vi "host.vi"() -> ()   [LabVIEW 2017]
panel:
  in  "Plot Color":u32(colorbox)=16715776
  in  "Grid Color":u32(colorbox)
  in  "Visible Section":u16(ring)=8
  out "Polar Plot":picture
  in  "stop":bool
  out "data":dbl(graph)
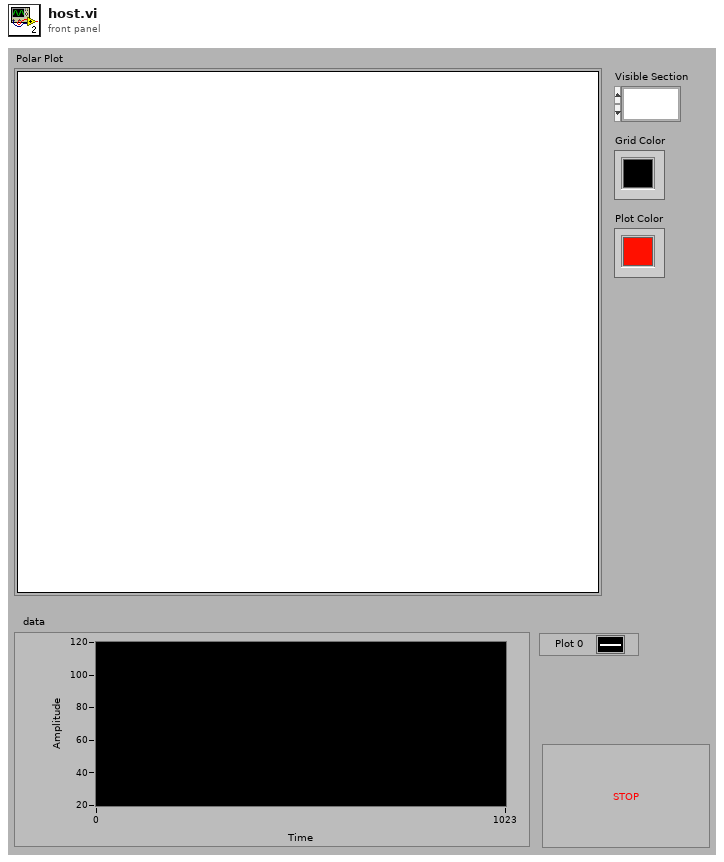
[diagram p1: front panel]
types:
  T1 = cluster{"maximum":dbl, "minimum":dbl, "clip to min":bool, "log?(F)":bool, "grid color":u32, "plot color":u32, "format and precision":cluster{"format":enum8{"Decimal", "Scientific", "Engineering", "Binary", "Octal", "Hex"}, "precision":u8}, "visible section":u16}
  T2 = typedef "LVBoundsTypeDef.ctl" = cluster{"Width":u32, "Height":u32}
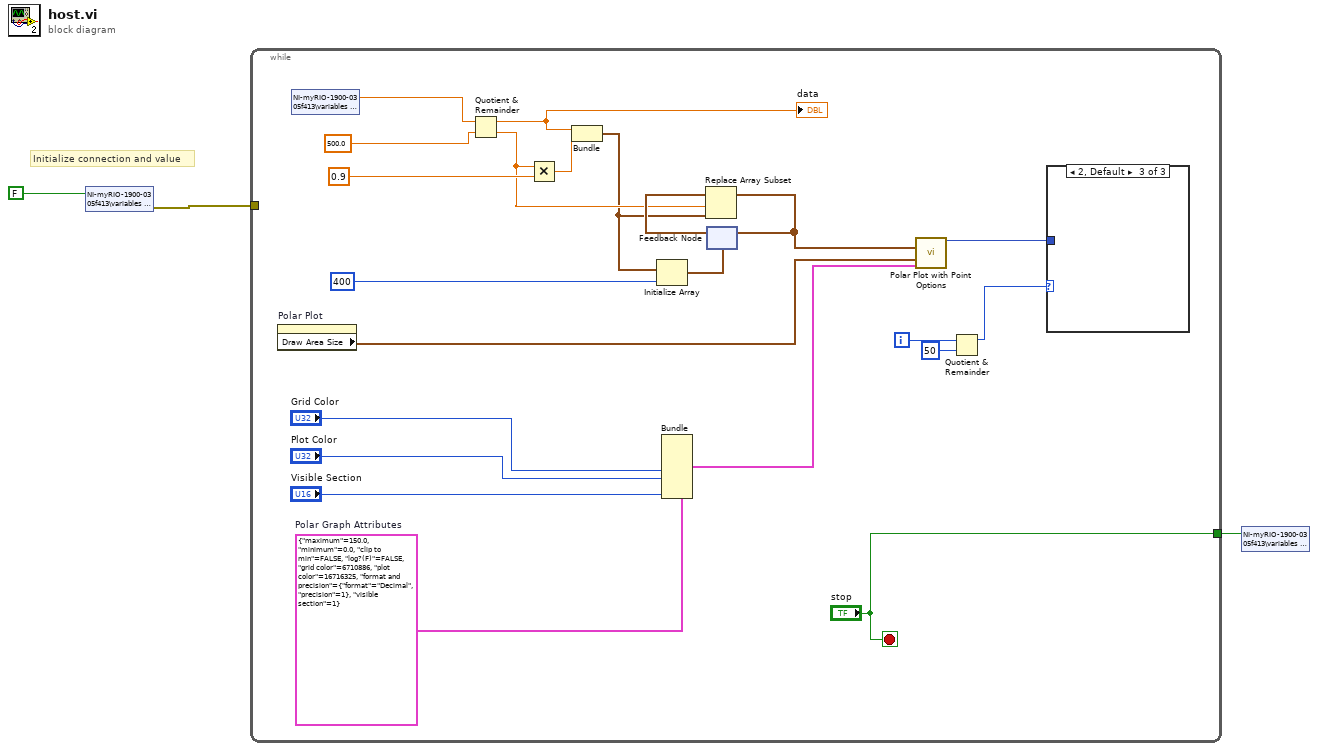
[diagram p0: block diagram]
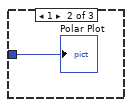
[diagram p3: hidden frame]
diagram:
  # "Initialize connection and value"
  n1 = shared-variable "NI-myRIO-1900-0305f413\\variables - network - RT.lvlib\\stop"(FALSE) -> (error out=w2:errorcluster)  [unwired: 1 in]
  n2 = while {
    tunnel: ["stop"] -> w3
    tunnel: w2 -> [_]
    i -> [w6]
    stop <- "stop" stop-if-true
    w11 = T1 {"maximum"=150.0, "minimum"=0.0, "clip to min"=FALSE, "log?(F)"=FALSE, "grid color"=6710886, "plot color"=16716325, "format and precision"={"format"=enum."Decimal", "precision"=1}, "visible section"=1}  # Polar Graph Attributes
    n3 = property on="Polar Plot" class="Pict"() -> ("Draw Area Size"=w22:T2)  [unwired: 2 in, 2 out]
    n4 = shared-variable "NI-myRIO-1900-0305f413\\variables - network - RT.lvlib\\data"() -> (w24:dbl)  [unwired: 1 in, 1 out]
    n5 = Quotient & Remainder(x=w24, y=500.0) -> (x-y*floor(x/y)=w15:dbl, floor(x/y)=w17:dbl)
    "data" <- w15
    n6 = Multiply(x=w17, y=0.9) -> (x*y=w19:dbl)
    n7 = Bundle(w15, w19) -> (w12:cluster{dbl, dbl})  [unwired: 1 in]
    n8 = Initialize Array(w12, 400 ("dimension size")) -> (w14:cluster{dbl, dbl}[])
    n9 = Bundle(cluster=w11, "grid color"="Grid Color", "plot color"="Plot Color", "visible section"="Visible Section") -> (w7:T1)  [unwired: 5 in]
    n10 = feedback #1(w14) -> (w18:cluster{dbl, dbl}[])
    n11 = Replace Array Subset(array=w18, new element=w12, index=w17) -> (w16:cluster{dbl, dbl}[])
    n12 = feedback-in #1(w16) -> ()
    n13 = call <vilib>:"Polar Plot with Point Options.vi"("data array [mag, phase (deg)]"=w16, "dimensions (w,h)"=w22, "polar attributes"=w7) -> ("new picture"=w21:picture)  [unwired: 12 in]
    n14 = Quotient & Remainder(x=w6, y=50) -> (x-y*floor(x/y)=w4:i32)  [unwired: 1 out]
    n15 = case shown="2, Default" w4 {
      tunnel: w21 -> [_ w26 _]
      frame 0 {
      }
      frame 1 {
        "Polar Plot" <- w26
      }
      frame 2, Default {
      }
    }
  }
  n16 = shared-variable "NI-myRIO-1900-0305f413\\variables - network - RT.lvlib\\stop"(w3) -> ()  [unwired: 1 in, 1 out]
